vi "Magnet Limits.vi"(0 "instrument.PPMS2":refnum<class "instrument.PPMS2.lvclass">, 5 "Helium (%)":dbl, 7 "Target Field (Oe)":dbl, 9 "Mode":T1, 11 "error in (no error)":errorcluster) -> (4 "instrument.PPMS2 out":refnum<class "instrument.PPMS2.lvclass">, 8 "Limited Field (Oe)":dbl, 10 "Mode out":T1, 15 "error out":errorcluster)   [LabVIEW 2019, in "instrument.PPMS2.lvclass"]
uses:
  instrument.PPMS2.lvclass
  <userlib>/LevyLab/Instrument Framework/Instrument Types/Cryostat/Typedefs/Magnet Mode--Enum.ctl
  <userlib>/LevyLab/Instrument Framework/Instrument Types/Cryostat/Instrument.Cryostat.lvclass
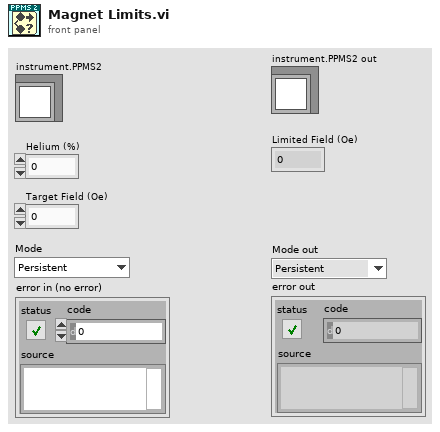
[diagram p1: front panel]
types:
  T1 = typedef "Instrument.Cryostat.lvclass/Magnet Mode--Enum.ctl" = enum16{"Persistent", "Driven"}
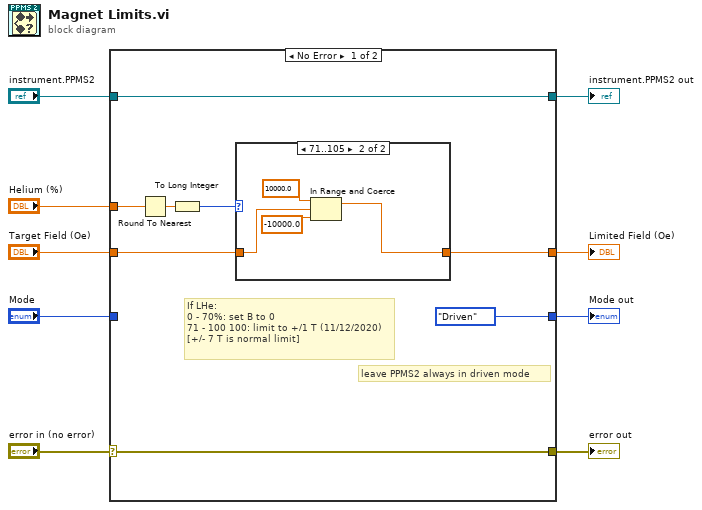
[diagram p0: block diagram]
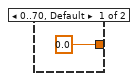
[diagram p2: hidden frame]
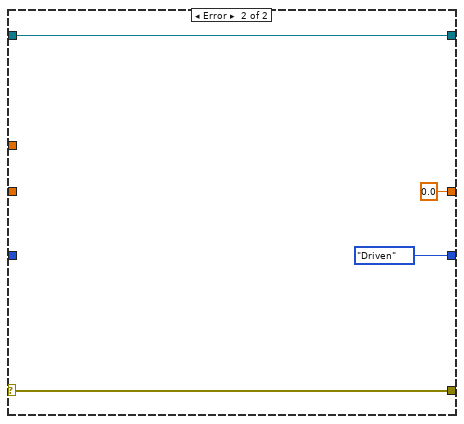
[diagram p3: hidden frame]
diagram:
  n1 = case shown="No Error" "error in (no error)" {
    selector: "error in (no error)" -> [w16 w26]
    tunnel: "Target Field (Oe)" -> [w11 _]
    tunnel: [w10 0.0 ("upper limit")] -> w2
    tunnel: "instrument.PPMS2" -> [w17 w25]
    tunnel: [w17 w25] -> w6
    tunnel: [w16 w26] -> w5
    tunnel: [Magnet_Mode--Enum."Driven" ("Mode") Magnet_Mode--Enum."Driven" ("Mode")] -> w3
    tunnel: "Mode" -> [_ _]
    tunnel: "Helium (%)" -> [w14 _]
    frame No Error {
      # "If LHe:\n0 - 70%: set B to 0\n71 - 100 100: limit to +/1 T (11/12/2020)\n[+/- 7 T is normal limit]"
      # "leave PPMS2 always in driven mode"
      n2 = Round To Nearest(number=w14) -> (nearest integer value=w13:dbl)
      n3 = To Long Integer(number=w13) -> (32bit integer=w12:i32)
      n4 = case shown="71..105" w12 {
        tunnel: w11 -> [_ w22]
        tunnel: [0.0 ("upper limit") w19] -> w10
        frame 0..70, Default {
        }
        frame 71..105 {
          n5 = In Range and Coerce(upper limit=10000.0, x=w22, lower limit=-10000.0) -> (coerced(x)=w19:dbl)  [unwired: 1 out]
        }
      }
    }
    frame Error {
    }
  }
  "Limited Field (Oe)" <- w2
  "instrument.PPMS2 out" <- w6
  "Mode out" <- w3
  "error out" <- w5
